vi "CommandDynamixelPosition.vi"(10 "NotifierReff":T1, 11 "VISA resource name":refnum<visa-resource-name>) -> (0 "Error out":errorcluster)   [LabVIEW 2013]
uses:
  Data/TypeDefs/Notifiers.ctl
  Data/TypeDefs/UTM Location.ctl
  Data/TypeDefs/Sail Set Suggestions.ctl
  Data/TypeDefs/Rudder Set Suggestions.ctl
  Data/TypeDefs/OverrideInformation.ctl
  Data/TypeDefs/OverrideMode.ctl
  Data/TypeDefs/MotorSetup.ctl
  Data/TypeDefs/DynamixelSetupInfo.ctl
  Data/TypeDefs/AirmarStatus.ctl
  Data/TypeDefs/HardwareOnline.ctl
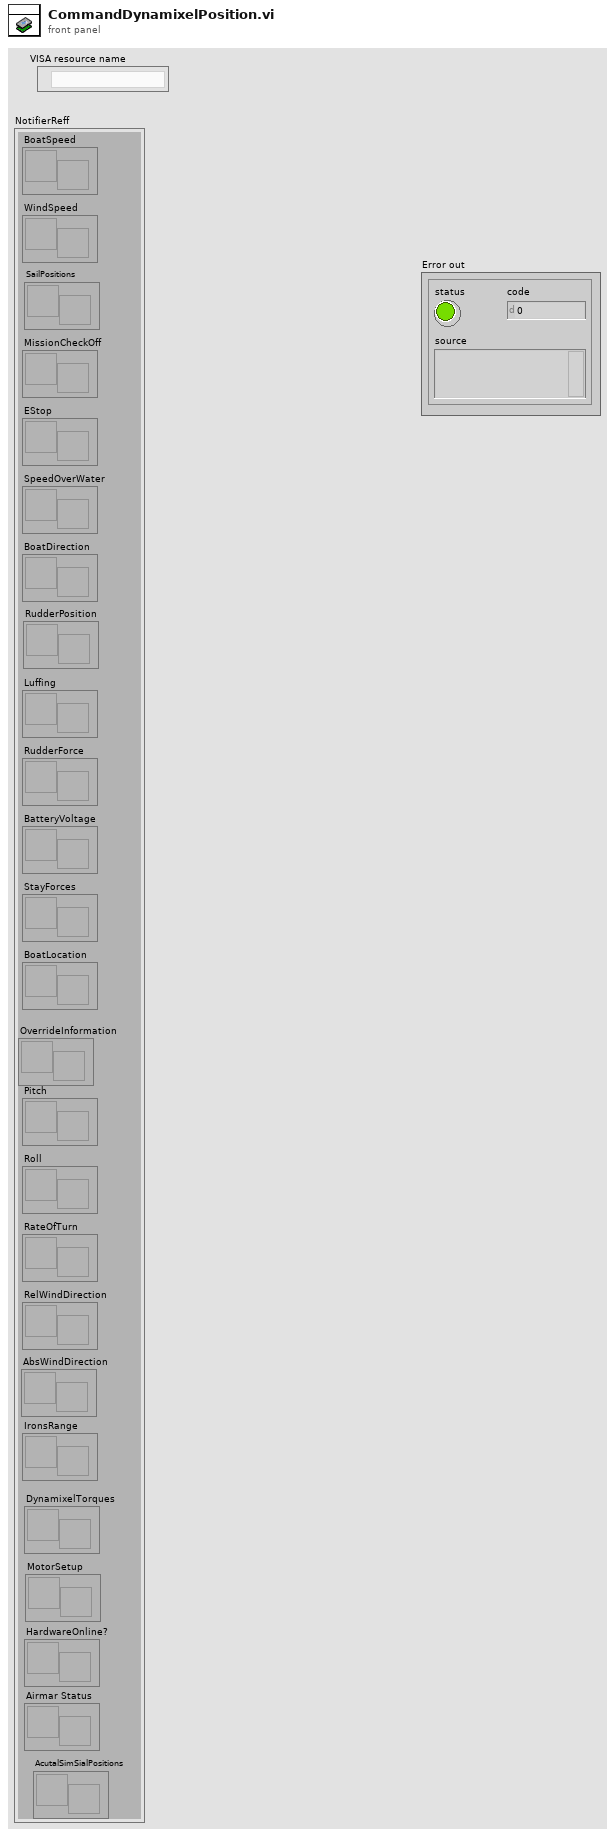
[diagram p1: front panel]
types:
  T1 = typedef "Notifiers.ctl" = cluster{"BoatSpeed":refnum<notifier>, "WindSpeed":refnum<notifier>, "MissionCheckOff":refnum<notifier>, "EStop":refnum<notifier>, "SpeedOverWater":refnum<notifier>, "BoatDirection":refnum<notifier>, "Luffing":refnum<notifier>, "RudderForce":refnum<notifier>, "BatteryVoltage":refnum<notifier>, "StayForces":refnum<notifier>, "BoatLocation":refnum<notifier>, "Pitch":refnum<notifier>, "Roll":refnum<notifier>, "RateOfTurn":refnum<notifier>, "RelWindDirection":refnum<notifier>, "SailPositions":refnum<notifier>, "RudderPosition":refnum<notifier>, "IronsRange":refnum<notifier>, "AbsWindDirection":refnum<notifier>, "OverrideInformation":refnum<notifier>, "DynamixelTorques":refnum<notifier>, "MotorSetup":refnum<notifier>, "Airmar Status":refnum<notifier>, "HardwareOnline?":refnum<notifier>, "AcutalSimSialPositions":refnum<notifier>}
  T2 = typedef "MotorSetup.ctl" = cluster{"Main Dynamixel Set Data":T3, "Rudder Dynamixel Set Data":T3, "Jib Dynamixel Set Data":T3}
  T3 = typedef "DynamixelSetupInfo.ctl" = cluster{"Lower Winch Bound":dbl, "Upper Winch Bound":dbl, "Reverse Winch Direction?":bool, "Dynamixel Cycle Number":i32}
  T4 = typedef "Sail Set Suggestions.ctl" = cluster{"MainSailSuggestion":dbl, "JibSailSuggestion":dbl}
  T5 = typedef "Rudder Set Suggestions.ctl" = dbl
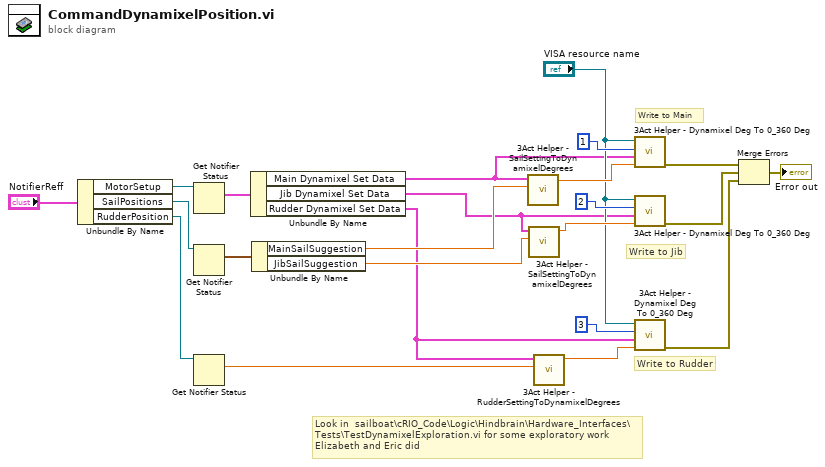
[diagram p0: block diagram]
diagram:
  # "Look in  sailboat\\cRIO_Code\\Logic\\Hindbrain\\Hardware_Interfaces\\Tests\\TestDynamixelExploration.vi for some exploratory work Elizabeth and Eric did"
  # "Write to Rudder"
  # "Write to Jib"
  # "Write to Main"
  n1 = Unbundle By Name("NotifierReff") -> ("MotorSetup"=w20:refnum<notifier>, "SailPositions"=w22:refnum<notifier>, "RudderPosition"=w16:refnum<notifier>)
  n2 = Get Notifier Status(notifier=w20) -> (current notification=w19:T2)  [unwired: 1 in, 4 out]
  n3 = Get Notifier Status(notifier=w22) -> (current notification=w21:T4)  [unwired: 1 in, 4 out]
  n4 = Get Notifier Status(notifier=w16) -> (current notification=w15:T5)  [unwired: 1 in, 4 out]
  n5 = Unbundle By Name(w19) -> ("Main Dynamixel Set Data"=w6:T3, "Jib Dynamixel Set Data"=w1:T3, "Rudder Dynamixel Set Data"=w7:T3)
  n6 = Unbundle By Name(w21) -> ("MainSailSuggestion"=w18:dbl, "JibSailSuggestion"=w17:dbl)
  n7 = call "3Act Helper - SailSettingToDynamixelDegrees.vi"("SailSuggestion"=w18, "Dynamixel Set Data"=w6) -> ("Dynamixel Angle"=w11:dbl)  [unwired: 9 in]
  n8 = call "3Act Helper - SailSettingToDynamixelDegrees.vi"("SailSuggestion"=w17, "Dynamixel Set Data"=w1) -> ("Dynamixel Angle"=w10:dbl)  [unwired: 9 in]
  n9 = call "3Act Helper - RudderSettingToDynamixelDegrees.vi"("Suggested Rudder Setpoint"=w15, "Dynamixel Set Data"=w7) -> ("Dynamixel Angle"=w8:dbl)  [unwired: 9 in]
  n10 = call "3Act Helper - Dynamixel Deg To 0_360 Deg.vi"("Dynamixel Setpoint In (deg)"=w11, "Dynamixel Set Data"=w6, "Motor ID"=u8 1 ("Motor ID (0)"), "VISA resource name"="VISA resource name") -> ("Error out"=w5:errorcluster)  [unwired: 7 in]
  n11 = call "3Act Helper - Dynamixel Deg To 0_360 Deg.vi"("Dynamixel Setpoint In (deg)"=w10, "Dynamixel Set Data"=w1, "Motor ID"=u8 2 ("Motor ID (0)"), "VISA resource name"="VISA resource name") -> ("Error out"=w4:errorcluster)  [unwired: 7 in]
  n12 = call "3Act Helper - Dynamixel Deg To 0_360 Deg.vi"("Dynamixel Setpoint In (deg)"=w8, "Dynamixel Set Data"=w7, "Motor ID"=u8 3 ("Motor ID (0)"), "VISA resource name"="VISA resource name") -> ("Error out"=w3:errorcluster)  [unwired: 7 in]
  n13 = Merge Errors(w5, w4, w3) -> (→"Error out":errorcluster)
